vi "Write DAQ FIFO.vi"(6 "FIFO Timestamps":T2, 8 "error in (no error)":errorcluster, 9 "Timeout (ms)":i32, 10 "Data In":T1[](array[typedef]), 11 "CIFChannels in":refnum<class "CIFChannels.lvclass">) -> (0 "error out":errorcluster, 1 "timed out?":bool, 2 "Data Out":T1[](array[typedef]), 3 "CIFChannels out":refnum<class "CIFChannels.lvclass">)   [LabVIEW 2021, in "CIFChannels.lvclass"]
uses:
  CIFChannels.lvclass
  ChannelCommon/typedef/TimeStamps.ctl
  CIFChannels.lvclass/CIFChannels.ctl
  ChannelCommon/typedef/Errors.ctl
  <vilib>/CIF Foundation/CIF Utilities/Errors/Append Error Location.vi
  ChannelCommon/ChannelCommon.lvlib
  ChannelCommon/typedef/Datatype Waveform.ctl
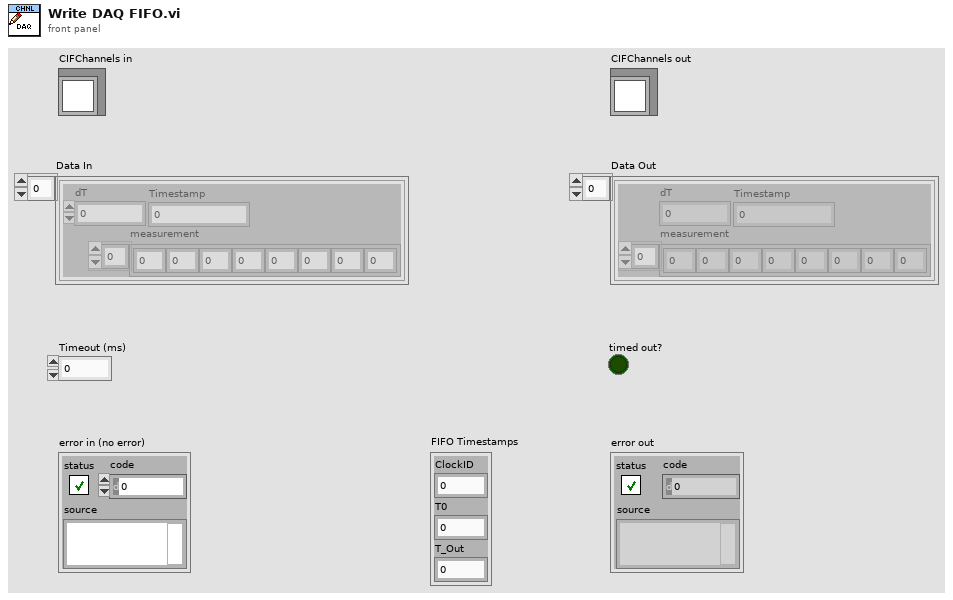
[diagram p1: front panel]
types:
  T1 = typedef "ChannelCommon.lvlib/Datatype Waveform.ctl" = cluster{"measurement":dbl[], "dT":dbl, "Timestamp":i64}
  T2 = typedef "ChannelCommon.lvlib/TimeStamps.ctl" = cluster{"ClockID":u8, "T0":i64, "T_Out":i64}
  T3 = typedef "ChannelCommon.lvlib/Errors.ctl" = enum16{"gRPC Server Not Found", "Duplicate Channel", "Missing Channel", "Incorrect Type", "Flatten Error", "Unflatten Data", "Channel Length", "Plugin Connection", "gRPC Server Connection", "FIFO Unflatten", "Required Override", "Remove Not Found"}
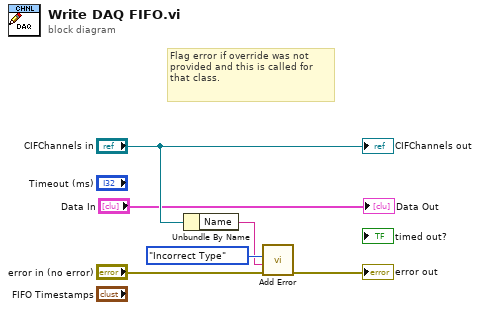
[diagram p0: block diagram]
diagram:
  # "Flag error if override was not provided and this is called for that class."
  n1 = Unbundle By Name("CIFChannels in") -> ("Name"=w2:string)
  n2 = call "Add Error.vi"("error in (no error)"="error in (no error)", "String to Append"=w2, "Error"=Errors."Incorrect Type") -> ("error out"=→"error out":errorcluster)  [unwired: 8 in]
  "CIFChannels out" <- "CIFChannels in"
  "Data Out" <- "Data In"
